vi "AlliGator Create Series Subfolders.vi"(8 "error in (no error)":errorcluster, 9 "Image Root String Separator (-)":string="-", 10 "pattern":string="*.png", 11 "Path":path) -> (0 "error out":errorcluster, 1 "Subfolder Paths":path[](array[path]), 2 "Sorted Subfolder Names":string[](array[string]), 3 "dup directory path":path, 4 "# Files":i32[](array[numeric]), 5 "Files in the Root Folder":string[](array[string]), 6 "Same # Files?":bool)   [LabVIEW 2021, in "AlliGator Files.lvlib"]
doc: "Sorts image files into folders of images (to handle early flat data structure generated by Pi Imaging SPAD512S device)."
uses:
  AlliGator Files.lvlib
  c9f14ad0-bdb9-48b7-805b-12724326120b.vi
  fe3d2969-a5f6-4b40-b7d1-1904744f1c3d.vi
  f3351217-9857-4bfd-98b4-4a43117e57ea.vi
  <userlib>/_OpenG.lib/array/array.llb/Delete Elements from 1D Array (String)__ogtk.vi
  <vilib>/Comparison/Less/Less Functor/Less Functor.lvclass
  <userlib>/_OpenG.lib/file/file.llb/openg_file.lvlib
  <userlib>/_OpenG.lib/array/array.llb/openg_array.lvlib
panel:
  out "# Folders":i32
  # "see the AlliGator License on the block diagram (Ctrl+E or Window:Show Block Diagram)"
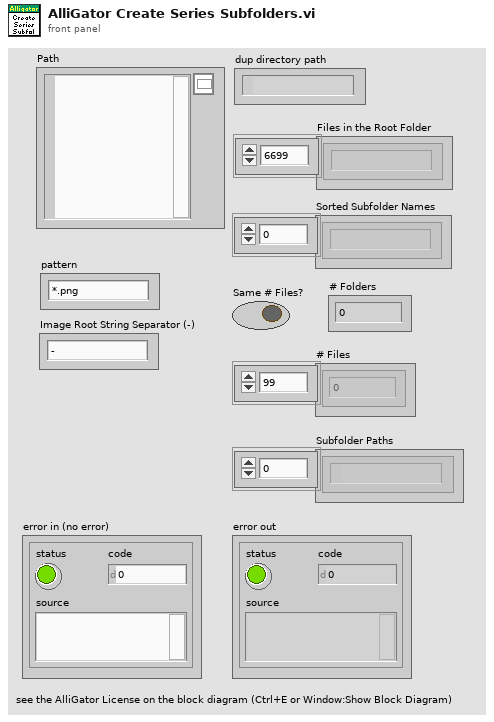
[diagram p1: front panel]
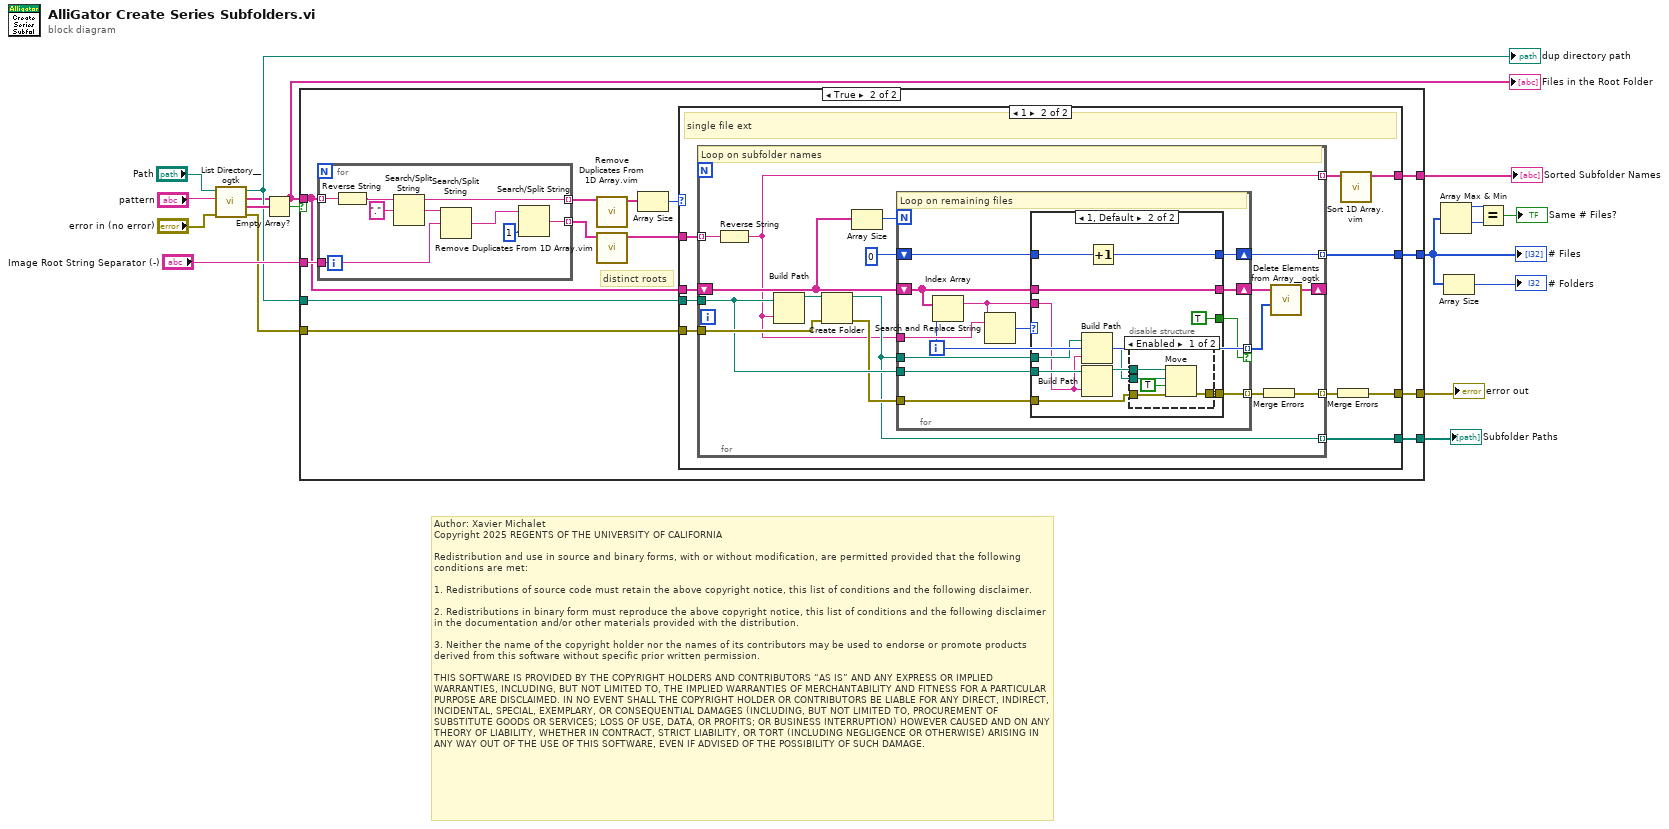
[diagram p0: block diagram]
diagram:
  # "Author: Xavier Michalet\nCopyright 2025 REGENTS OF THE UNIVERSITY OF CALIFORNIA\n\nRedistribution and use in source and binary forms, with or without modification, are permitted provided that the following conditions are met:\n\n1. Redistributions of source code must retain the above copyright notice, this list of conditions and the following disclaimer.\n\n2. Redistributions in binary form must reproduce the above copyright notice, this list of conditions and the following disclaimer in the documentation and/or other materials provided with the distribution.\n\n3. Neither the name of the copyright holder nor the names of its contributors may be used to endorse or promote products derived from this software without specific prior written permission.\n\nTHIS SOFTWARE IS PROVIDED BY THE COPYRIGHT HOLDERS AND CONTRIBUTORS “AS IS” AND ANY EXPRESS OR IMPLIED WARRANTIES, INCLUDING, BUT NOT LIMITED TO, THE IMPLIED WARRANTIES OF MERCHANTABILITY AND FITNESS FOR A PARTICULAR PURPOSE ARE DISCLAIMED. IN NO EVENT SHALL THE COPYRIGHT HOLDER OR CONTRIBUTORS BE LIABLE FOR ANY DIRECT, INDIRECT, INCIDENTAL, SPECIAL, EXEMPLARY, OR CONSEQUENTIAL DAMAGES (INCLUDING, BUT NOT LIMITED TO, PROCUREMENT OF SUBSTITUTE GOODS OR SERVICES; LOSS OF USE, DATA, OR PROFITS; OR BUSINESS INTERRUPTION) HOWEVER CAUSED AND ON ANY THEORY OF LIABILITY, WHETHER IN CONTRACT, STRICT LIABILITY, OR TORT (INCLUDING NEGLIGENCE OR OTHERWISE) ARISING IN ANY WAY OUT OF THE USE OF THIS SOFTWARE, EVEN IF ADVISED OF THE POSSIBILITY OF SUCH DAMAGE."
  n1 = call <userlib>:"List Directory__ogtk.vi"("error in (no error)"="error in (no error)", "pattern"="pattern", "directory path"="Path") -> ("error out"=w10:errorcluster, "directory names"=w15:string[], "file names"=w1:string[], "dup directory path"=w11:path)  [unwired: 1 in]
  "dup directory path" <- w11
  "Files in the Root Folder" <- w1
  n2 = Empty Array?(array=w15) -> (empty?=w14:bool)
  n3 = case shown="True" w14 {
    tunnel: w1 -> [_ w24]
    tunnel: "Image Root String Separator (-)" -> [_ w28]
    tunnel: w11 -> [_ w26]
    tunnel: w10 -> [w18 w25]
    tunnel: [w18 w23] -> w9
    tunnel: [_ w21] -> w6
    tunnel: [_ w20] -> w7
    tunnel: [_ w19] -> w2
    frame False {
    }
    frame True {
      # "distinct roots"
      n4 = for {
        tunnel: w24 -> [w100] mode=indexing
        tunnel: [w97] -> w31 mode=indexing
        tunnel: [w95] -> w27 mode=indexing
        tunnel: w28 -> [w92]
        n5 = Reverse String(1:w100) -> (0:w99:string)
        n6 = Search/Split String(string=w99, search string/char (-)="." ("search string")) -> (substring before match=w97:string, match + rest of string=w94:string)  [unwired: 1 in, 1 out]
        n7 = Search/Split String(string=w94, search string/char (-)=w92) -> (match + rest of string=w93:string)  [unwired: 1 in, 2 out]
        n8 = Search/Split String(string=w93, offset (0)=1) -> (match + rest of string=w95:string)  [unwired: 1 in, 2 out]
      }
      n9 = call "Remove Duplicates From 1D Array.vim"("array"=w31) -> ("array with duplicates removed"=w29:string[])  [unwired: 10 in]
      n10 = call "Remove Duplicates From 1D Array.vim"("array"=w27) -> ("array with duplicates removed"=w22:string[])  [unwired: 10 in]
      n11 = Array Size(array=w29) -> (size(s)=w30:i32)
      n12 = case shown="1" w30 {
        tunnel: w22 -> [_ w42]
        tunnel: w26 -> [_ w41]
        tunnel: w25 -> [w32 w40]
        tunnel: w24 -> [_ w39]
        tunnel: [w32 w37] -> w23
        tunnel: [_ w36] -> w21
        tunnel: [_ w35] -> w20
        tunnel: [_ w33] -> w19
        frame 0, Default {
          # "multiple ext: give up"
        }
        frame 1 {
          # "single file ext"
          n13 = for {
            tunnel: w42 -> [w58] mode=indexing
            tunnel: w41 -> [w55]
            tunnel: w40 -> [w56]
            shift-right: [w45] -> _
            shift-left: w39 -> [w51]
            tunnel: [w52] -> w38 mode=indexing
            tunnel: [w48] -> w36 mode=indexing
            tunnel: [w47] -> w35 mode=indexing
            tunnel: [w43] -> w34 mode=indexing
            # "Loop on subfolder names"
            n14 = Reverse String(1:w58) -> (0:w43:string)
            n15 = Build Path(base path=w55, name or relative path=w43) -> (appended path=w57:path)
            n16 = Create Folder(path (use dialog)=w57, error in=w56) -> (created path=w47:path, error out=w54:errorcluster)  [unwired: 1 in, 1 out]
            n17 = Array Size(array=w51) -> (size(s)=w50:i32)
            n18 = for {
              N: w50 -> [_]
              shift-right: [w64] -> w46
              shift-left: w51 -> [w70]
              tunnel: w43 -> [w71]
              tunnel: w47 -> [w69]
              tunnel: w55 -> [w68]
              tunnel: w54 -> [w66]
              tunnel: [w65] -> w53 mode=indexing
              shift-right: [w62] -> w48
              shift-left: 0 -> [w63]
              tunnel: [w60] -> w44 mode=indexing if=w59
              i -> [w60]
              # "Loop on remaining files"
              n19 = Index Array(array=w70, index=w60) -> (element=w67:string)
              n20 = Search and Replace String(input string=w67, search string=w71) -> (number of replacements=w61:i32)  [unwired: 6 in, 3 out]
              n21 = case shown="1, Default" w61 {
                tunnel: w70 -> [w74 w85]
                tunnel: [w74 w85] -> w64
                tunnel: w69 -> [_ w82]
                tunnel: w68 -> [_ w84]
                tunnel: w67 -> [_ w81]
                tunnel: w66 -> [w73 w79]
                tunnel: [w73 w78] -> w65
                tunnel: w63 -> [w72 w77]
                tunnel: [w72 w76] -> w62
                tunnel: [_ TRUE] -> w59
                frame 0 {
                  # "different root name"
                }
                frame 1, Default {
                  n22 = Build Path(base path=w82, name or relative path=w81) -> (appended path=w80:path)
                  n23 = Build Path(base path=w84, name or relative path=w81) -> (appended path=w83:path)
                  n24 = Increment(x=w77) -> (x+1=w76:i32)
                  n25 = disable-structure shown="Enabled" {
                    disable-tunnel: w83 -> [w90 _]
                    disable-tunnel: w80 -> [w89 _]
                    disable-tunnel: w79 -> [w88 w91]
                    disable-tunnel: [w87 w91] -> w78
                    frame Enabled {
                      n26 = Move(source path=w90, error in=w88, 9:TRUE ("overwrite (F)"), 10:w89) -> (error out=w87:errorcluster)  [unwired: 1 in, 2 out]
                    }
                    frame Disabled {
                    }
                  }
                }
              }
            }
            n27 = Merge Errors(w53) -> (w52:errorcluster)
            n28 = call-poly <userlib>:"Delete Elements from Array__ogtk.vi"("indices"=w44, "array"=w46) -> ("array w/ subset deleted"=w45:string[])  [unwired: 8 in, 1 out]
          }
          n29 = Merge Errors(w38) -> (w37:errorcluster)
          n30 = call "Sort 1D Array.vim"("unsorted array"=w34) -> ("sorted array"=w33:string[])  [unwired: 10 in]
        }
      }
    }
  }
  "Sorted Subfolder Names" <- w2
  "# Files" <- w6
  "error out" <- w9
  "Subfolder Paths" <- w7
  n31 = Array Max & Min(array=w6) -> (max value=w5:i32, min value=w4:i32)  [unwired: 2 out]
  n32 = Array Size(array=w6) -> (size(s)=→"# Folders":i32)
  n33 = Equal?(x=w5, y=w4) -> (x = y?=→"Same # Files?":bool)
